vi "PS Get Limits.vi"(0 "PS Communication Port":refnum<visa-resource-name>) -> (1 "Setpoint":dbl format="%.2f", 2 "Max Current":dbl format="%.2f", 3 "Slew Limits":cluster{dbl, dbl, dbl} {"?" format="%.2f"; "?" format="%.2f"; "?" format="%.2f"}, 4 "dup VISA Resource Name":refnum<visa-resource-name>, 5 "Slew Rate":dbl format="%.2f", 6 "Cell":u32, 7 "error out":errorcluster)   [LabVIEW 2021]
uses:
  Serial Support VISA.llb/Serial Actions.ctl
  Serial Support VISA.llb/Serial port parmeters.ctl
  PS Comm Globals.vi
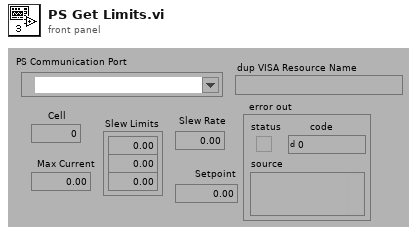
[diagram p1: front panel]
types:
  T1 = typedef "Serial Actions.ctl" = enum16{"Init", "Break", "Clear Buffer", "Write", "Read", "N Bytes", "Lock", "Unlock", "Close"}
  T2 = typedef "Serial port parmeters.ctl" = cluster{"flow control":enum16{"None", "XON/XOFF", "RTS/CTS"}, "baud rate":u32, "data bits":u16, "Stop Bits":u16, "parity (0:none)":enum16{"None", "Odd", "Even", "Mark", "Space"}, "Transmit Buffer Size":u32, "Receive Buffer Size":u32}
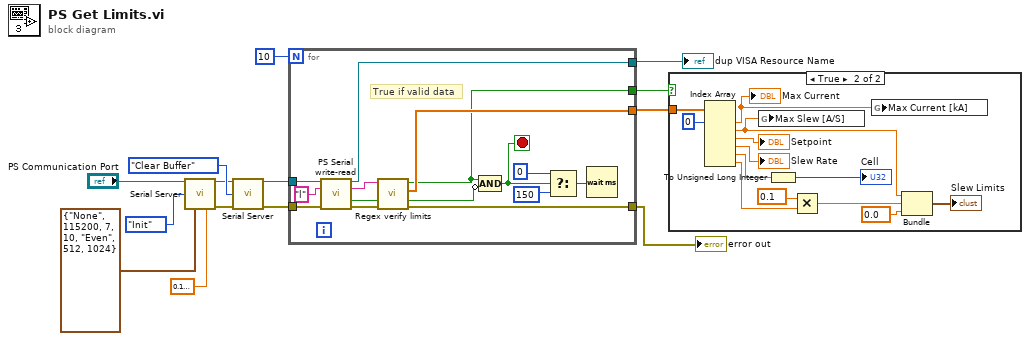
[diagram p0: block diagram]
diagram:
  n1 = call "Serial Server.vi"("VISA Resource Name"="PS Communication Port", "Action"=Serial_Actions."Init", "Port Parameters"=T2 {"flow control"=enum."None", "baud rate"=115200, "data bits"=7, "Stop Bits"=10, "parity (0:none)"=enum."Even", "Transmit Buffer Size"=512, "Receive Buffer Size"=1024}, "Timeout Limit(sec)"=sgl 0.1) -> ("dup VISA Resource Name"=w4:refnum<visa-resource-name>, "error out"=w2:errorcluster)  [unwired: 7 in, 3 out]
  n2 = call "Serial Server.vi"("VISA Resource Name"=w4, "Action"=Serial_Actions."Clear Buffer", "error in (no error)"=w2) -> ("dup VISA Resource Name"=w3:refnum<visa-resource-name>, "error out"=w1:errorcluster)  [unwired: 8 in, 3 out]
  n3 = for {
    N: 10 ("y") -> [_]
    tunnel: [w16] -> w11
    tunnel: [w17] -> w13
    tunnel: w1 -> [w26]
    tunnel: w3 -> [w27]
    tunnel: [w25] -> w12
    tunnel: [w15] -> w6
    stop <- w23 stop-if-true
    # "True if valid data"
    n4 = call "PS Serial write-read.vi"("VISA Resource Name"=w27, "String To Send"="l", "error in (no error)"=w26) -> ("dup VISA Resource Name"=w25:refnum<visa-resource-name>, "Serial Read"=w19:string, "Timeout"=w24:bool, "error out"=w18:errorcluster)  [unwired: 8 in, 1 out]
    n5 = call "Regex verify limits.vi"("error in"=w18, "input string"=w19) -> ("error out"=w17:errorcluster, "Data out"=w16:dbl[], "Valid data"=w15:bool)  [unwired: 7 in]
    n6 = Compound Arithmetic op=AND(w15, invert w24) -> (w23:bool)
    n7 = Select(t=u32 0, s=w23, f=u32 150 ("milliseconds to wait")) -> (s? t:f=w22:u32)
    n8 = Wait (ms)(milliseconds to wait=w22) -> ()  [unwired: 1 out]
  }
  "error out" <- w13
  "dup VISA Resource Name" <- w12
  n9 = case shown="True" w6 {
    tunnel: w11 -> [_ w36]
    frame False {
    }
    frame True {
      n10 = Index Array(array=w36, index #1=0) -> (element #1=w35:dbl, element #2=w34:dbl, element #3=→"Setpoint":dbl, element #4=→"Slew Rate":dbl, element #5=w31:dbl, element #6=w30:dbl)  [unwired: 5 in]
      "Max Current" <- w35
      n11 = global write "PS Comm Globals.vi" "Max Slew [A/S]"(w34) -> ()
      n12 = To Unsigned Long Integer(number=w31) -> (unsigned 32bit integer=→"Cell":u32)
      n13 = Multiply(x=0.1, y=w30) -> (x*y=w39:dbl)
      n14 = global write "PS Comm Globals.vi" "Max Current [kA]"(w35) -> ()
      n15 = Bundle(w34, w39, 0.0) -> (→"Slew Limits":cluster{dbl, dbl, dbl})  [unwired: 1 in]
    }
  }
